vi "PhotonTrackedTarget_GetCameraToTarget.vi"(11 "TrackedTarget":T4={"Yaw"=0.0, "Pitch"=0.0, "Area"=0.0, "Skew"=0.0, "TargetCorners"=[], "CameraToTarget"={"TRANSLATION"={"X"=0.0, "Y"=0.0}, "ROTATION"={"VALUE"=0.0, "COS"=1.0, "SIN"=0.0}}} {"CameraToTarget"."ROTATION"."SIN" format="%13.4f"; "CameraToTarget"."ROTATION"."COS" format="%13.4f"; "CameraToTarget"."ROTATION"."VALUE" format="%13.4f"; "CameraToTarget"."TRANSLATION"."Y" format="%14.3f"; "CameraToTarget"."TRANSLATION"."X" format="%14.3f"}) -> (3 "CameraToTarget":T1={"TRANSLATION"={"X"=0.0, "Y"=0.0}, "ROTATION"={"VALUE"=0.0, "COS"=1.0, "SIN"=0.0}} {"ROTATION"."SIN" format="%13.4f"; "ROTATION"."COS" format="%13.4f"; "ROTATION"."VALUE" format="%13.4f"; "TRANSLATION"."Y" format="%14.3f"; "TRANSLATION"."X" format="%14.3f"})   [LabVIEW 2019, in "PhotonVisionLib.lvlib"]
doc: "Get CameraToTarget Transform2d from Tracked Target\n\nInputs:\n - TrackedTarget -- Parsed TrackedTarget cluster.\n\nOutputs:\n - CameraToTarget -- Camera to Target Transform2d"
uses:
  TypeDef/PhotonTrackedTargetType.ctl
  TypeDef/TargetCornerType.ctl
  <vilib>/Rock Robotics/WPI/ThirdParty/JAS_Junk/TrajLib/TRANSFORM2D.ctl
  <vilib>/Rock Robotics/WPI/ThirdParty/JAS_Junk/TrajLib/TRANSLATION2D.ctl
  <vilib>/Rock Robotics/WPI/ThirdParty/JAS_Junk/TrajLib/ROTATION2D.ctl
  PhotonVisionLib.lvlib
  <vilib>/Rock Robotics/WPI/ThirdParty/JAS_Junk/TrajLib/Trajectory_Library.lvlib
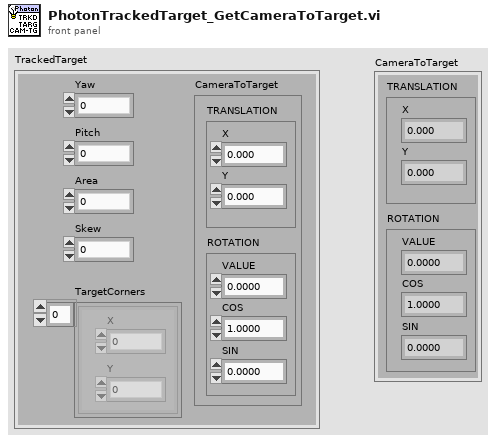
[diagram p1: front panel]
types:
  T1 = typedef "Trajectory_Library.lvlib/TRANSFORM2D.ctl" = cluster{"TRANSLATION":T2, "ROTATION":T3}
  T2 = typedef "Trajectory_Library.lvlib/TRANSLATION2D.ctl" = cluster{"X":dbl, "Y":dbl}
  T3 = typedef "Trajectory_Library.lvlib/ROTATION2D.ctl" = cluster{"VALUE":dbl, "COS":dbl, "SIN":dbl}
  T4 = typedef "PhotonVisionLib.lvlib/PhotonTrackedTargetType.ctl" = cluster{"Yaw":dbl, "Pitch":dbl, "Area":dbl, "Skew":dbl, "TargetCorners":T5[], "CameraToTarget":T1}
  T5 = typedef "PhotonVisionLib.lvlib/TargetCornerType.ctl" = cluster{"X":dbl, "Y":dbl}
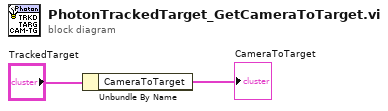
[diagram p0: block diagram]
diagram:
  n1 = Unbundle By Name("TrackedTarget") -> ("CameraToTarget"=→"CameraToTarget":T1)
